vi "cluster_v4.vi"() -> ()   [LabVIEW 2009]
panel:
  in  "Array":u8[](array[numeric])=[255, 0, 255, 0, 255, 0, 255, 0, 255, 0, 255, 0, 0, 0, 0, 255, 255, 0]
  in  "Coloana cu care se incepe":dbl
  in  "Numarul de octeti luati impreuna":i32=1
  in  "Latimea unei pozitii":dbl=2.0
  out "Digital Waveform Graph":cluster{dbl, dbl, u8[], i32}(graph)={0.0, 2.0, [255, 0, 255, 0, 255, 0, 255, 0, 255, 0, 255, 0, 0, 0, 0, 255, 255, 0], 1}
  # "Exista 16 coloane. Pe fiecare coloana se afiseaza in binar \ncate un numar din Array"
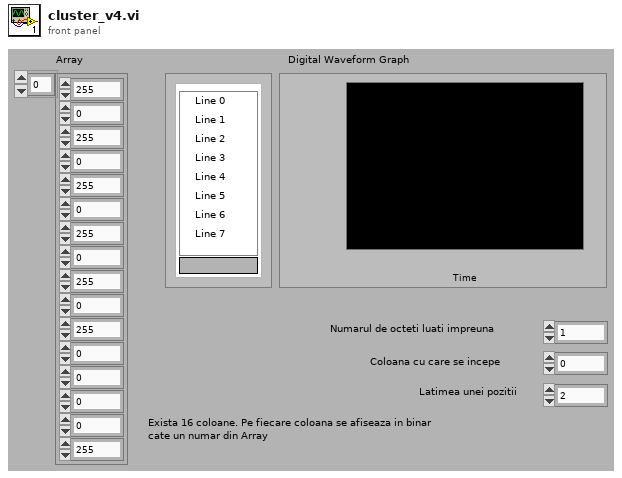
[diagram p1: front panel]
types:
  T1 = cluster{"Coloana cu care se incepe":dbl, "Latimea unei pozitii":dbl, "Array":u8[], "Numarul de octeti luati impreuna":i32}
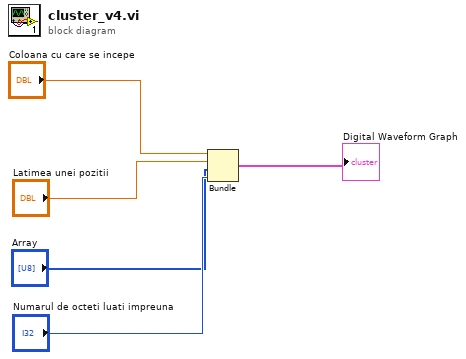
[diagram p0: block diagram]
diagram:
  n1 = Bundle("Coloana cu care se incepe"="Coloana cu care se incepe", "Latimea unei pozitii"="Latimea unei pozitii", "Array"="Array", "Numarul de octeti luati impreuna"="Numarul de octeti luati impreuna") -> (→"Digital Waveform Graph":T1)  [unwired: 1 in]
